vi "Channel selector.vi"(10 "CH2":bool, 11 "CH1":bool) -> (3 "Array":string[](array[string]))   [LabVIEW 2018]
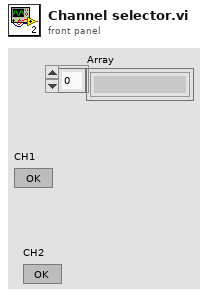
[diagram p1: front panel]
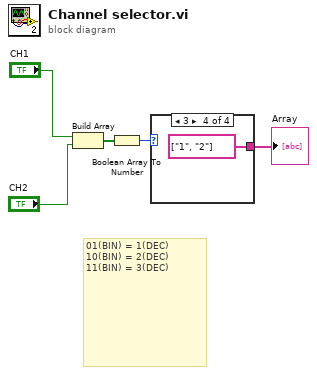
[diagram p0: block diagram]
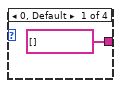
[diagram p2: hidden frame]
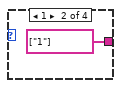
[diagram p3: hidden frame]
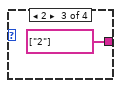
[diagram p4: hidden frame]
diagram:
  # "01(BIN) = 1(DEC)\n10(BIN) = 2(DEC)\n11(BIN) = 3(DEC)"
  n1 = Build Array("CH1", "CH2") -> (w1:bool[])
  n2 = Boolean Array To Number(Boolean array=w1) -> (number=w4:u32)
  n3 = case shown="3" w4 {
    tunnel: [string[] [] string[] ["1"] string[] ["2"] string[] ["1", "2"]] -> w5
    frame 0, Default {
    }
    frame 1 {
    }
    frame 2 {
    }
    frame 3 {
    }
  }
  "Array" <- w5
